vi "FRCts20_Backend_Test_Stats_GET.vi"(8 "error in (no error)":errorcluster) -> (0 "error out":errorcluster, 1 "Time (ms)":u32, 2 "Status":string, 5 "Success":bool)   [LabVIEW 2014, in "FRCts20_Backend_TestCode.lvlib"]
uses:
  FRCts20_Backend_TestCode.lvlib
  FRCts20_Backend_API/FRCts20_Backend_API_Stats.ctl
  ESP Engine/source/VI Source/TypeDefs/FRCts20_EspEngine_RequestPerHour_Line.ctl
  ESP Engine/source/VI Source/TypeDefs/FRCts20_EspEngine_SwUsage_Pie.ctl
  ESP Engine/source/VI Source/TypeDefs/FRCts20_EspEngine_AdvancedComponents_Bar.ctl
  FRCts20_Backend_API/FRCts20_Backend_API_Command_Stats.ctl
  FRCts20_Backend_API/FRCts20_Backend_API_Stats.vi
  FRCts20_Backend_API/FRCts20_Backend_API.lvlib
  ESP Engine/source/VI Source/FRCts20_EspEngine.lvlib
panel:
  out "Statistics Out":T1
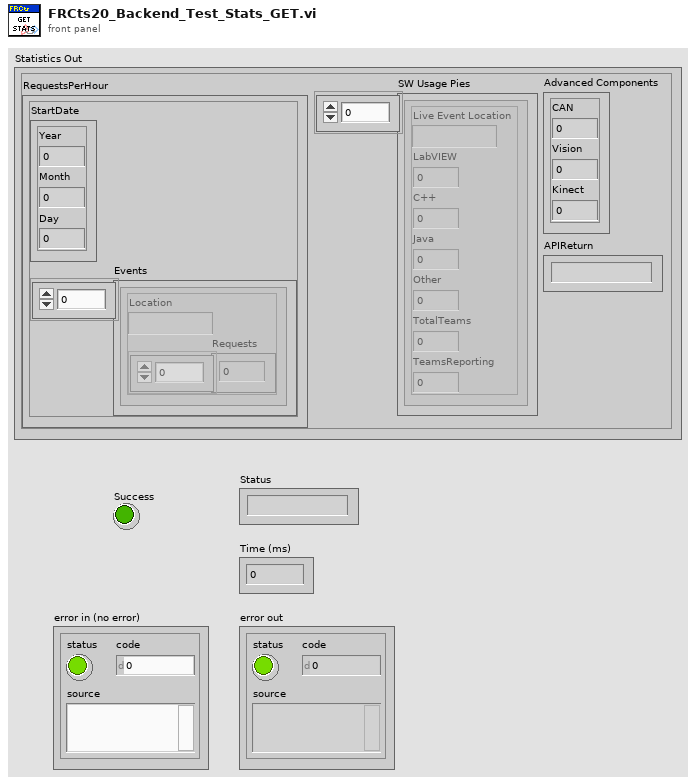
[diagram p1: front panel]
types:
  T1 = typedef "FRCts20_Backend_API.lvlib/FRCts20_Backend_API_Stats.ctl" = cluster{"RequestsPerHour":T2, "SW Usage Pies":T3, "Advanced Components":T4, "APIReturn":string}
  T2 = typedef "FRCts20_EspEngine.lvlib/FRCts20_EspEngine_RequestPerHour_Line.ctl" = cluster{"StartDate":cluster{"Year":i32, "Month":i32, "Day":i32}, "Events":cluster{"Location":string, "Requests":i32[]}[]}
  T3 = typedef "FRCts20_EspEngine.lvlib/FRCts20_EspEngine_SwUsage_Pie.ctl" = cluster{"Live Event Location":string, "LabVIEW":dbl, "C++":dbl, "Java":dbl, "Other":dbl, "TotalTeams":i32, "TeamsReporting":i32}[]
  T4 = typedef "FRCts20_EspEngine.lvlib/FRCts20_EspEngine_AdvancedComponents_Bar.ctl" = cluster{"CAN":i32, "Vision":i32, "Kinect":i32}
  T5 = typedef "FRCts20_Backend_API.lvlib/FRCts20_Backend_API_Command_Stats.ctl" = string
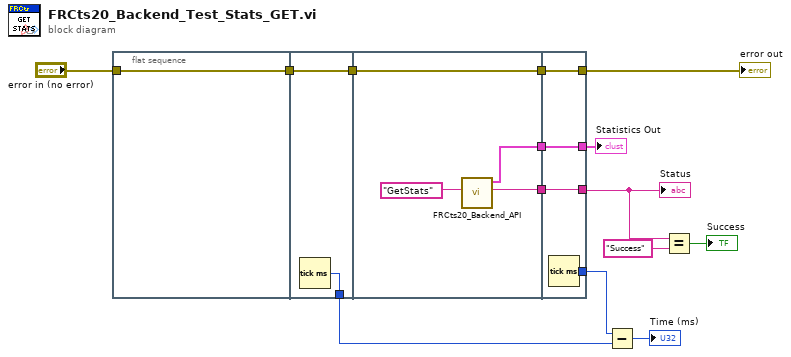
[diagram p0: block diagram]
diagram:
  n1 = flat-sequence {
    tunnel: "error in (no error)" -> [w15]
    tunnel: [w15] -> w14
    tunnel: [w17] -> w7
    tunnel: [w16] -> w13
    tunnel: w14 -> [w16]
    tunnel: [w21] -> w12
    tunnel: [w20] -> w11
    tunnel: [w19] -> w10
    tunnel: w13 -> [w19]
    tunnel: w12 -> [w25]
    tunnel: w11 -> [w24]
    tunnel: [w25] -> w4
    tunnel: [w24] -> w1
    tunnel: [w23] -> w6
    tunnel: [w22] -> w9
    tunnel: w10 -> [w22]
    frame #0 {
    }
    frame #1 {
      n2 = Tick Count (ms)() -> (millisecond timer value=w17:u32)
    }
    frame #2 {
      n3 = call-poly "FRCts20_Backend_API.vi"("Command"=T5 "GetStats") -> ("Status"=w21:string, "Statistics Out"=w20:T1)  [unwired: 8 in, 1 out]
    }
    frame #3 {
      n4 = Tick Count (ms)() -> (millisecond timer value=w23:u32)
    }
  }
  n5 = Subtract(x=w6, y=w7) -> (x-y=→"Time (ms)":u32)
  n6 = Equal?(x=w4, y="Success") -> (x = y?=→"Success":bool)
  "error out" <- w9
  "Status" <- w4
  "Statistics Out" <- w1
